vi "LS340-TempTester.vi"(11 "error in (no error)":errorcluster) -> ()   [LabVIEW 2012]
doc: "This VI was designed to demonstrate typical usage of sub VIs containing the more common 218 functions. The VI Initializes the instrument, calls the Application Temperature Monitor VI, and then closes the instrument. The Application Temperature Monitor VI first configures the input group and input to be read using the LSCI 218 Config input.vi. Time is then provided for the instrument to configure the input group and input. Finally, the selected input is read."
uses:
  <instrlib>/Lake Shore Cryotronics 340/Lake Shore Cryotronics 340.lvlib
panel:
  in  "SelectComPort":refnum<visa-resource-name>
  out "error out":errorcluster={"status"=FALSE, "code"=1073676418, "source"="VISA Close in MON_LS218_Init.vi->LS218-TempTester.vi"}
  out "VISA Out":refnum<visa-resource-name>="ASRL5::INSTR"
  out "*IDN?":string="LSCI,MODEL218S,219303,020602\r"
  # "Firt Select \"SelectComPort\" , then Click Run.  To stop GUI,  click \" Press to EXIT\""
  # "LakeShore 340 Temperature Tester"
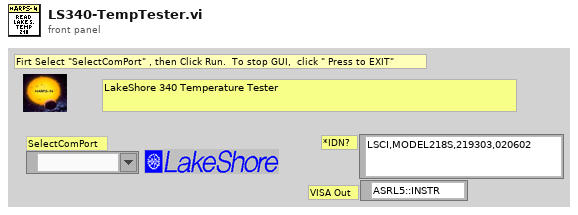
[diagram p1: front panel]
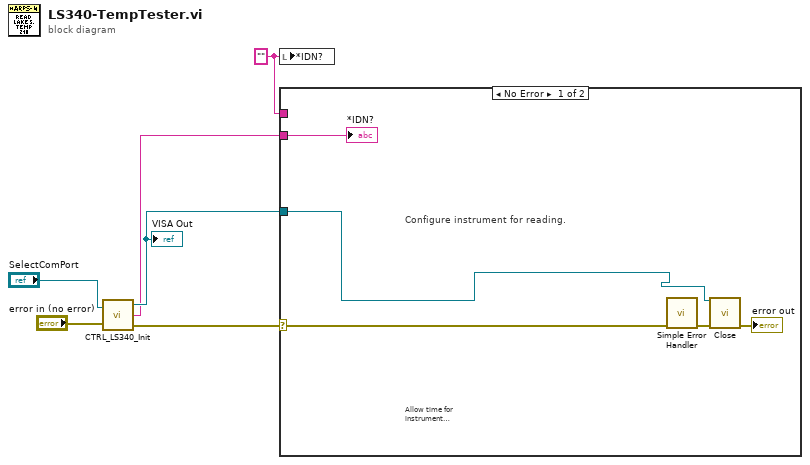
[diagram p0: block diagram]
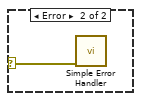
[diagram p2: hidden frame]
diagram:
  w5 = "" ("reply")
  n1 = call "CTRL_LS340_Init.vi"("error in (no error)"="error in (no error)", "found VISA"="SelectComPort") -> ("error out"=w1:errorcluster, "Reply"=w2:string, "VISA Out"=w3:refnum<visa-resource-name>)
  "VISA Out" <- w3
  n2 = local write "*IDN?"(w5) -> ()
  n3 = case shown="No Error" w1 {
    selector: w1 -> [w8 w12]
    tunnel: w3 -> [w7 _]
    tunnel: w2 -> [w9 _]
    tunnel: w5 -> [_ _]
    frame No Error {
      # "Allow time for instrument \nto initialize."
      # "Configure instrument for reading."
      n4 = call <vilib>:"Simple Error Handler.vi"("error in (no error)"=w8) -> ("error out"=w11:errorcluster)  [unwired: 4 in, 4 out]
      n5 = call <instrlib>:"Close.vi"("VISA resource name"=w7, "error in (no error)"=w11) -> ("error out"=→"error out":errorcluster)  [unwired: 13 in]
      "*IDN?" <- w9
    }
    frame Error {
      n6 = call <vilib>:"Simple Error Handler.vi"("error in (no error)"=w12) -> ()  [unwired: 4 in, 5 out]
    }
  }
